vi "myRIO_BRig_RT_TCP__buildStr_analogInput__PortA.vi"(10 "input_AI1":u16, 11 "input_AI0":u16) -> (3 "output_str_analogInput":string)   [LabVIEW 2014]
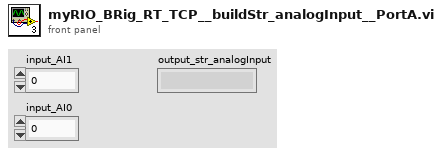
[diagram p1: front panel]
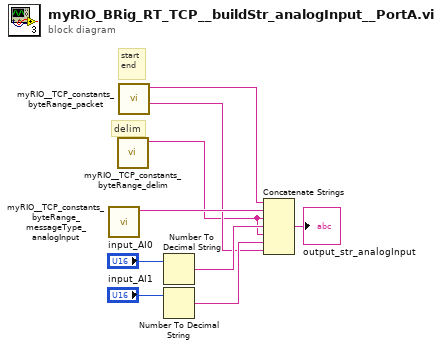
[diagram p0: block diagram]
diagram:
  # "start\nend"
  # "delim"
  n1 = call "myRIO__TCP_constants_byteRange_messageType_analogInput.vi"() -> ("output_analogInput_char"=w7:string)  [unwired: 10 in, 1 out]
  n2 = call "myRIO__TCP_constants_byteRange_delim.vi"() -> ("output_delim_char"=w2:string)  [unwired: 10 in, 1 out]
  n3 = call "myRIO__TCP_constants_byteRange_packet.vi"() -> ("output_end_char"=w3:string, "output_start_char"=w4:string)  [unwired: 8 in, 2 out]
  n4 = Number To Decimal String(number="input_AI0") -> (decimal integer string=w8:string)  [unwired: 1 in]
  n5 = Number To Decimal String(number="input_AI1") -> (decimal integer string=w9:string)  [unwired: 1 in]
  n6 = Concatenate Strings(w4, w7, w2, w8, w2, w9, w3) -> (→"output_str_analogInput":string)
